vi "[Template]_Static Write.vi"(8 "error in (no error)":errorcluster, 9 "Data":T1, 11 "Tag Name":string) -> (0 "error out":errorcluster)   [LabVIEW 2020, in "Current Value Table(Rebuild).lvlib"]
doc: "This VI will write the data associated with a single tag. This VI will only look up the tag index on the first call, or if the look-up resulted in an error. This VI has higher performance than the normal write function thanks to the removal of the name check."
uses:
  [Template]_Datatype.ctl
  Current Value Table(Rebuild).lvlib
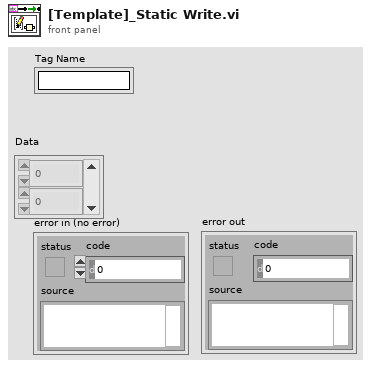
[diagram p1: front panel]
types:
  T1 = typedef "Current Value Table(Rebuild).lvlib/[Template]_Datatype.ctl" = i32[]
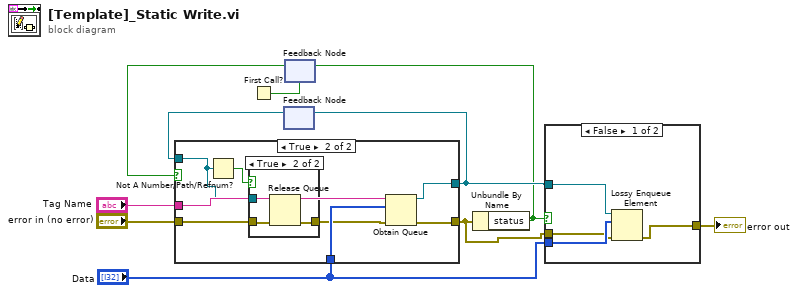
[diagram p0: block diagram]
diagram:
  n1 = First Call?() -> (First Call?: T/F=w4:bool)
  n2 = feedback #1() -> (w8:refnum<queue>)  [unwired: 1 in]
  n3 = feedback #2(w4) -> (w5:bool)
  n4 = case shown="True" w5 {
    tunnel: [w12 w20] -> w2
    tunnel: "error in (no error)" -> [w12 w15]
    tunnel: [w11 w18] -> w10
    tunnel: w8 -> [w11 w13]
    tunnel: "Tag Name" -> [_ w19]
    tunnel: "Data" -> [_ w17]
    frame False {
    }
    frame True {
      n5 = Not A Number/Path/Refnum?(number/path/refnum=w13) -> (NaN/Path/Refnum?=w16:bool)
      n6 = case shown="True" w16 {
        tunnel: w15 -> [w21 w23]
        tunnel: [w21 w24] -> w14
        tunnel: w13 -> [_ w22]
        frame False {
        }
        frame True {
          n7 = Release Queue(queue=w22, error in (no error)=w23) -> (error out=w24:errorcluster)  [unwired: 1 in, 2 out]
        }
      }
      n8 = Obtain Queue(name (unnamed)=w19, element data type=w17, error in (no error)=w14) -> (queue out=w18:refnum<queue>, error out=w20:errorcluster)  [unwired: 2 in, 1 out]
    }
  }
  n9 = feedback-in #1(w10) -> ()
  n10 = Unbundle By Name(w2) -> ("status"=w6:bool)
  n11 = feedback-in #2(w6) -> ()
  n12 = case shown="False" w6 {
    tunnel: w10 -> [w25 _]
    tunnel: "Data" -> [w28 _]
    tunnel: w2 -> [w27 w29]
    tunnel: [w26 w29] -> w1
    frame False {
      n13 = Lossy Enqueue Element(queue=w25, element=w28, error in (no error)=w27) -> (error out=w26:errorcluster)  [unwired: 3 out]
    }
    frame True {
    }
  }
  "error out" <- w1
